vi "MGI Occurrence[] to String.vi"(7 "Add Column Header? (F)":bool, 8 "error in (no error)":errorcluster, 10 "Error[]":errorcluster[](array[cluster]), 11 "MGI Error Reporter Base In":refnum<class "MGI Error Reporter Base.lvclass">) -> (0 "error out":errorcluster, 2 "Delimited String":string, 3 "MGI Error Reporter Base Out":refnum<class "MGI Error Reporter Base.lvclass">)   [LabVIEW 2016, in "MGI Error Reporter Base.lvclass"]
doc: "Format the array of Error Occurrence into a string appropriate for the error log file. Child classes may override this VI and format the error log file as appropriate. This VI creates a tab delimited text line for each error occurrance.\n\nAuthored by Shawn Walpole\nsupport@mooregoodideas.com\nwww.mooregoodideas.com\n\nCopyright (c) 2013, Moore Good Ideas, Inc.\n\nAll rights reserved.\n\nRedistribution and use in source and binary forms, with or without modification, are permitted provided that the following conditions are met:\n\n * Redistributions of source code must retain the above copyright notice, this list of conditions and the following disclaimer.\n * Redistributions in binary form must reproduce the above copyright notice, this list of conditions and the following disclaimer in the documentation and/or other materials provided with the distribution.\n * Neither the name of Moore Good Ideas, Inc. nor the names of its contributors may be used to endorse or promote products derived from this software without specific prior written permission.\n\nTHIS SOFTWARE IS PROVIDED BY THE COPYRIGHT HOLDERS AND CONTRIBUTORS \"AS IS\" AND ANY EXPRESS OR IMPLIED WARRANTIES, INCLUDING, BUT NOT LIMITED TO, THE IMPLIED WARRANTIES OF MERCHANTABILITY AND FITNESS FOR A PARTICULAR PURPOSE ARE DISCLAIMED. IN NO EVENT SHALL THE COPYRIGHT OWNER OR CONTRIBUTORS BE LIABLE FOR ANY DIRECT, INDIRECT, INCIDENTAL, SPECIAL, EXEMPLARY, OR CONSEQUENTIAL DAMAGES (INCLUDING, BUT NOT LIMITED TO, PROCUREMENT OF SUBSTITUTE GOODS OR SERVICES; LOSS OF USE, DATA, OR PROFITS; OR BUSINESS INTERRUPTION) HOWEVER CAUSED AND ON ANY THEORY OF LIABILITY, WHETHER IN CONTRACT, STRICT LIABILITY, OR TORT (INCLUDING NEGLIGENCE OR OTHERWISE) ARISING IN ANY WAY OUT OF THE USE OF THIS SOFTWARE, EVEN IF ADVISED OF THE POSSIBILITY OF SUCH DAMAGE."
uses:
  <userlib>/_MGI/Error Reporter/MGI Error Reporter Base/MGI Error Reporter Base.lvclass
  <userlib>/_MGI/Error Reporter/MGI Error Reporter Base/MGI Error Reporter Base.lvclass/MGI Error Reporter Base.ctl
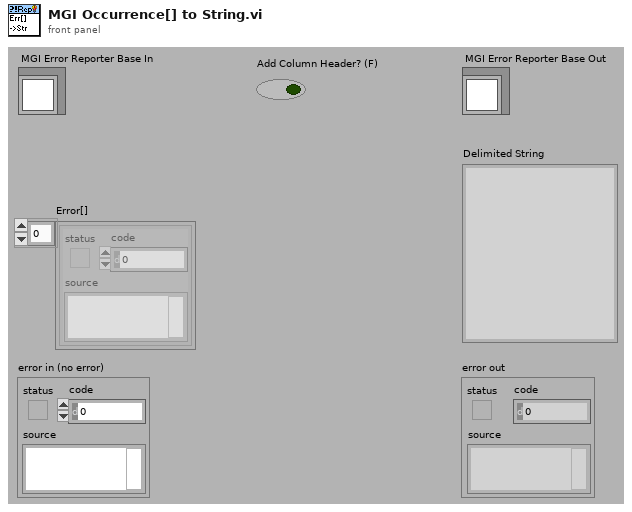
[diagram p1: front panel]
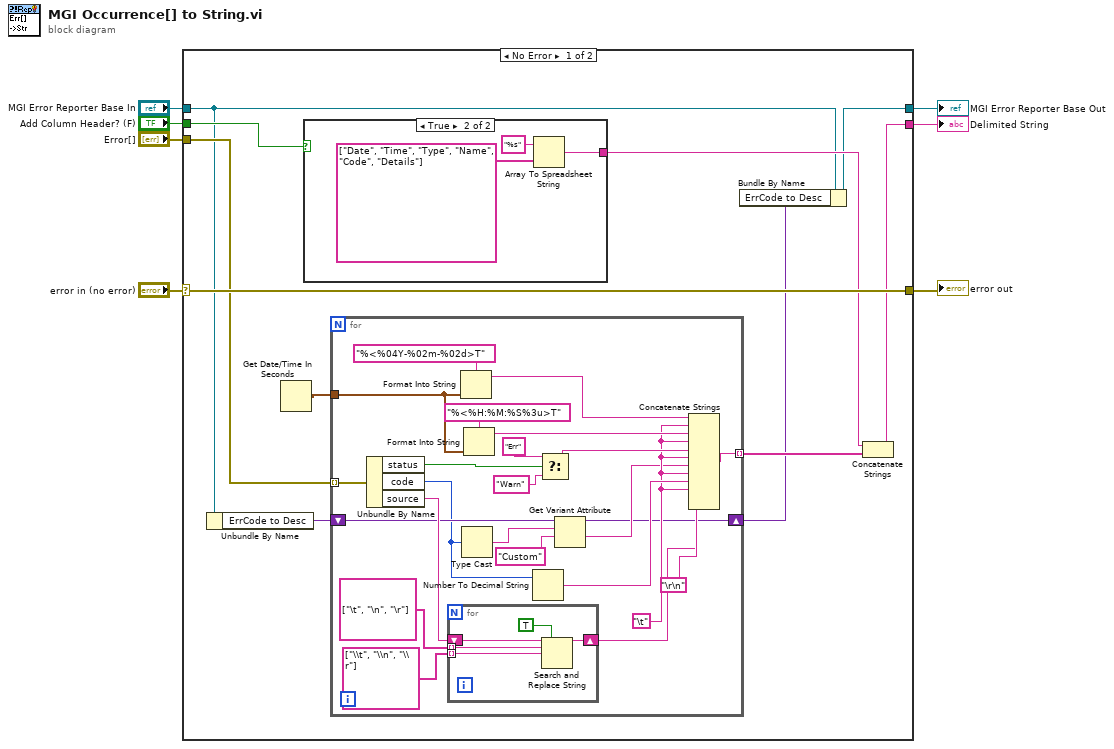
[diagram p0: block diagram]
diagram:
  n1 = case shown="No Error" "error in (no error)" {
    selector: "error in (no error)" -> [w18 w52]
    tunnel: [w18 w52] -> w6
    tunnel: [w10 w51] -> w4
    tunnel: "MGI Error Reporter Base In" -> [w11 w51]
    tunnel: "Error[]" -> [w17 _]
    tunnel: [w15 _] -> w3
    tunnel: "Add Column Header? (F)" -> [w14 _]
    frame No Error {
      n2 = Unbundle By Name(w11) -> ("ErrCode to Desc"=w12:variant)
      n3 = Get Date/Time In Seconds() -> (seconds since 1Jan1904=w8:timestamp)
      n4 = case shown="True" w14 {
        tunnel: [_ w19] -> w13
        frame False {
        }
        frame True {
          n5 = Array To Spreadsheet String(array=string[] ["Date", "Time", "Type", "Name", "Code", "Details"], 3:"%s" ("format string")) -> (spreadsheet string=w19:string)  [unwired: 1 out]
        }
      }
      n6 = for {
        tunnel: w17 -> [w45] mode=indexing
        tunnel: [w40] -> w16 mode=indexing
        shift-right: [w25] -> w9
        shift-left: w12 -> [w26]
        tunnel: w8 -> [w22]
        w34 = "\t"
        n7 = Unbundle By Name(w45) -> ("status"=w39:bool, "code"=w24:i32, "source"=w31:string)
        n8 = for {
          shift-right: [w50] -> w32
          shift-left: w31 -> [w49]
          tunnel: string[] ["\t", "\n", "\r"] -> [w47] mode=indexing
          tunnel: string[] ["\\t", "\\n", "\\r"] -> [w46] mode=indexing
          n9 = Search and Replace String(replace all?=TRUE ("replace all? (F)"), input string=w49, search string=w47, replace string=w46) -> (result string=w50:string)  [unwired: 1 in, 6 out]
        }
        n10 = Format Into String(format string="%<%04Y-%02m-%02d>T", w22) -> (resulting string=w42:string)  [unwired: 2 in, 1 out]
        n11 = Type Cast(x=w24) -> (*(type *) &x=w23:string)  [unwired: 1 out]
        n12 = Format Into String(format string="%<%H:%M:%S%3u>T", w22) -> (resulting string=w41:string)  [unwired: 2 in, 1 out]
        n13 = Number To Decimal String(number=w24) -> (decimal integer string=w35:string)  [unwired: 1 out]
        n14 = Select(t="Err", s=w39, f="Warn") -> (s? t:f=w36:string)
        n15 = Get Variant Attribute(Variant=w26, name=w23, default value (empty Variant)="Custom" ("name")) -> (duplicate Variant=w25:variant, value=w28:string)  [unwired: 1 in, 2 out]
        n16 = Concatenate Strings(w42, w34, w41, w34, w36, w34, w28, w34, w35, w34, w32, "\r\n") -> (w40:string)
      }
      n17 = Bundle By Name(cluster=w11, "ErrCode to Desc"=w9) -> (w10:refnum<class "MGI Error Reporter Base.lvclass">)
      n18 = Concatenate Strings(w13, w16) -> (w15:string)
    }
    frame Error {
    }
  }
  "error out" <- w6
  "MGI Error Reporter Base Out" <- w4
  "Delimited String" <- w3
